vi "chr63204A_CC_L1_read.vi"(8 "error in (no error)":errorcluster, 11 "VISA resource name":refnum<visa-resource-name>) -> (0 "error out":errorcluster, 2 "Value":dbl, 3 "VISA resource name out":refnum<visa-resource-name>)   [LabVIEW 2020]
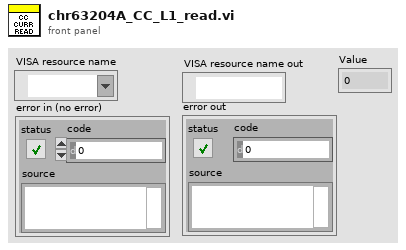
[diagram p1: front panel]
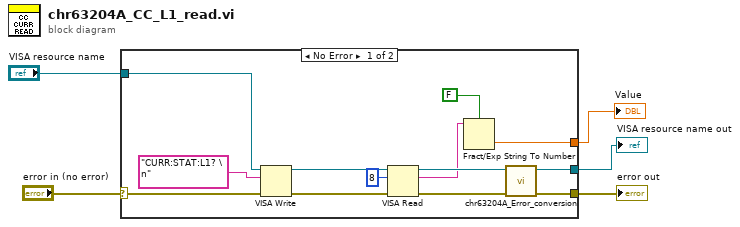
[diagram p0: block diagram]
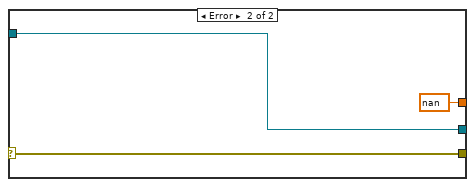
[diagram p2: hidden frame]
diagram:
  n1 = case shown="No Error" "error in (no error)" {
    selector: "error in (no error)" -> [w17 w20]
    tunnel: "VISA resource name" -> [w18 w21]
    tunnel: [w16 w21] -> w3
    tunnel: [w15 w20] -> w2
    tunnel: [w7 nan] -> w1
    frame No Error {
      n2 = VISA Write(VISA resource name=w18, write buffer="CURR:STAT:L1? \n" ("string"), error in (no error)=w17) -> (VISA resource name out=w13:refnum<visa-resource-name>, error out=w12:errorcluster)  [unwired: 1 out]
      n3 = VISA Read(VISA resource name=w13, byte count=u32 8, error in (no error)=w12) -> (VISA resource name out=w11:refnum<visa-resource-name>, read buffer=w8:string, error out=w10:errorcluster)  [unwired: 1 out]
      n4 = Fract/Exp String To Number(use system decimal point (T)=FALSE, string=w8) -> (number=w7:dbl)  [unwired: 2 in, 1 out]
      n5 = call "chr63204A_Error_conversion.vi"("error in (no error)"=w10, "VISA resource name"=w11) -> ("error out"=w15:errorcluster, "VISA resource name out"=w16:refnum<visa-resource-name>)  [unwired: 8 in]
    }
    frame Error {
    }
  }
  "VISA resource name out" <- w3
  "error out" <- w2
  "Value" <- w1
